vi "CRYTS Step Insert.vi"(10 "Steps":refnum<vi>, 11 "Tree Task SequenceIn":refnum<vi>) -> (3 "Tree Task Sequence Out":refnum<vi>)   [LabVIEW 2013]
uses:
  CRYSystem/Typedef Control/CRYStep.ctl
  CRYProject Editor Global.vi
  CRYMainGlobal.vi
panel:
  # "Insert new step into Project window."
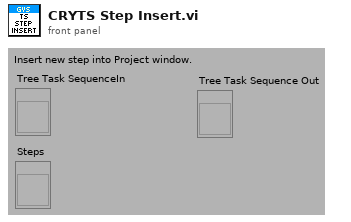
[diagram p1: front panel]
types:
  T1 = typedef "CRYTS.ctl" = cluster{"No.TS":u16, "TS File Path":path, "TS Name":string, "EditStepName":string, "Steps":T2[], "New State":bool, "Change State":bool, "Flattened CurveLib Data":string, "Document Data":string, "EditStepNo":u16, "Operator Start File":string, "Sequence Type":string, "Sequence Language":string}
  T2 = typedef "CRYStep.ctl" = cluster{"No.VI":i32, "Category":string, "StepName":string, "Seq setup flattened":string, "Comment":string, "Steps config.":bool[], "Jump config":i32[], "Start":dbl, "Increment":dbl, "Name":string, "Unit":string, "Y data":u16, "Y prefix":string, "Y dB ref":dbl, "Y unit":string, "Repeat State Array":cluster{"Start":dbl, "Increment":dbl, "Count":i32, "Num":i32}[]}
  T3 = cluster{"SourceRowNum":i32, "SourceCount":i32, "TargetRowNum":i32, "bResult":bool, "EditRowNum":i32}
  T4 = cluster{"Content":string, "Name":string, "Level":u32, "Category":string}[]
  T5 = cluster{"Content":string, "Name":string, "Level":u32, "Category":string}
  T6 = enum16{"Insert", "Remove", "Move up", "Move down"}
  T7 = cluster{"Start":dbl, "Increment":dbl, "Count":i32, "Num":i32}[]
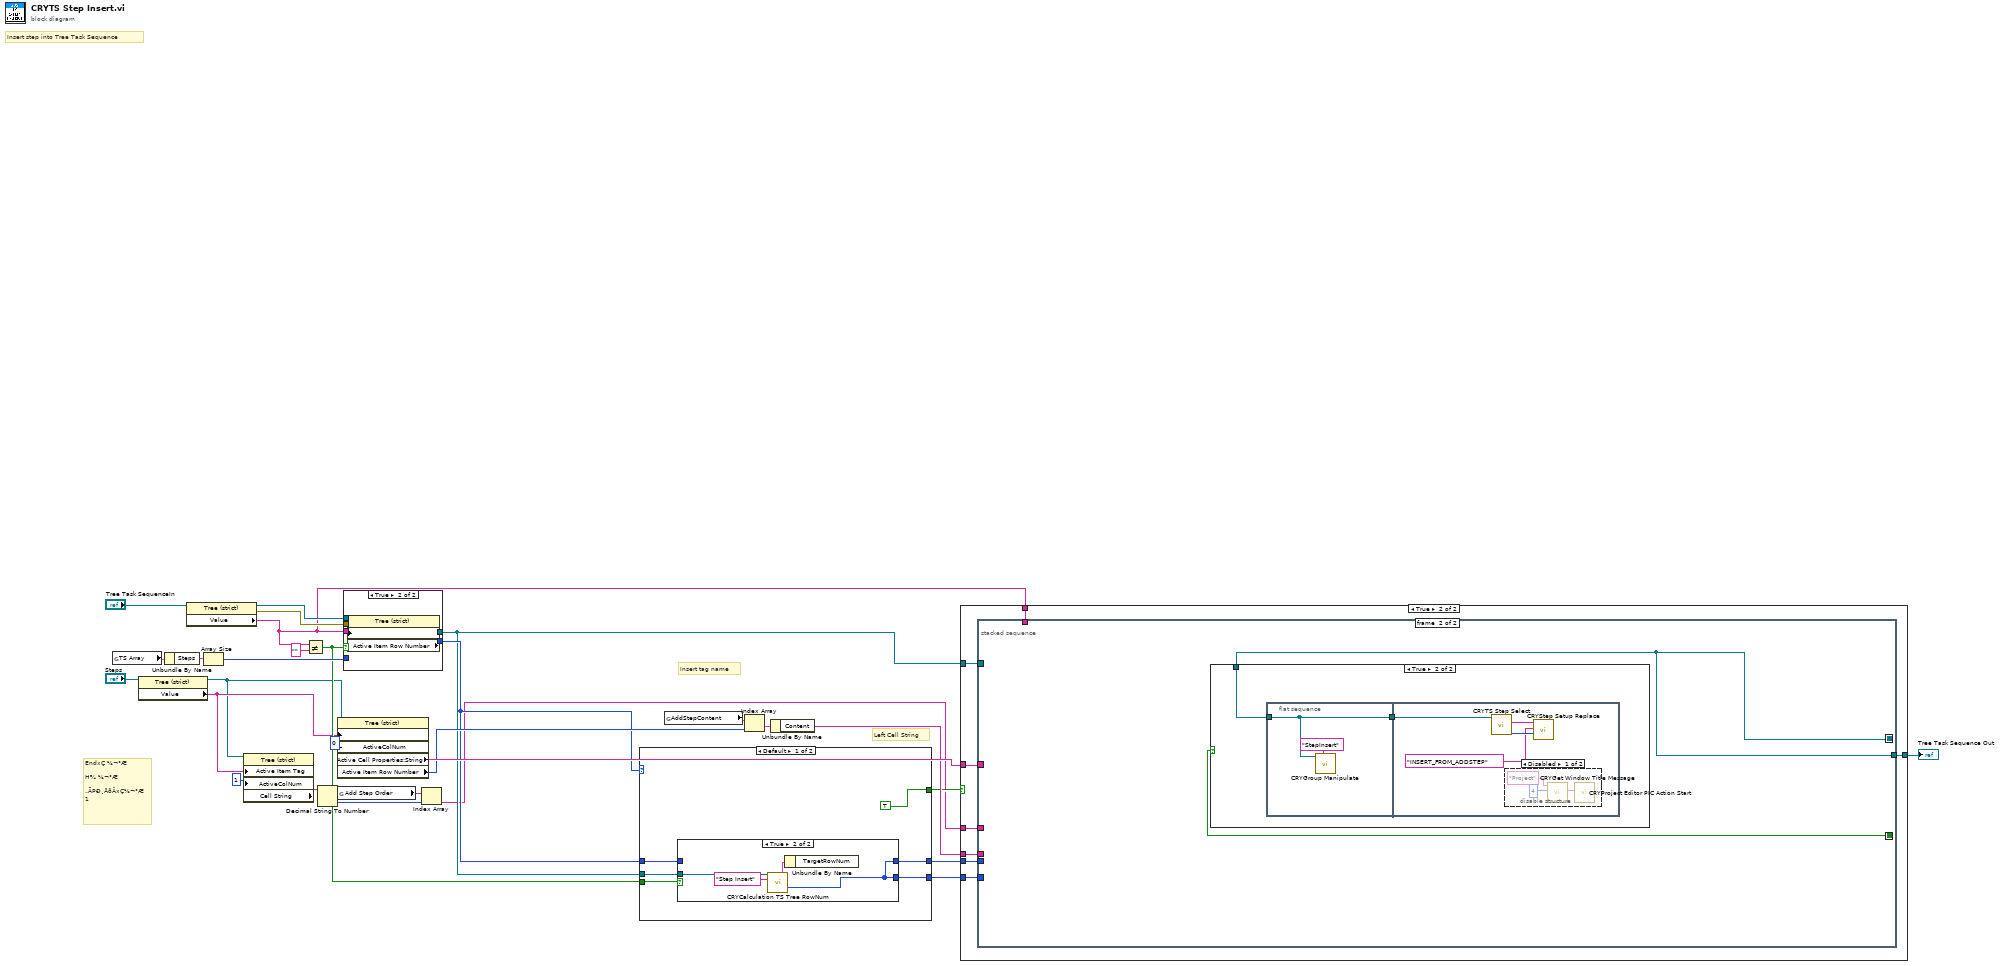
[diagram p0: block diagram]
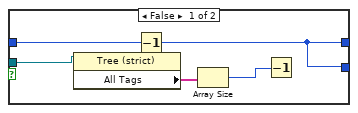
[diagram p2: hidden frame]
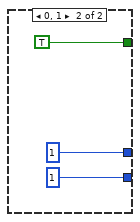
[diagram p3: hidden frame]
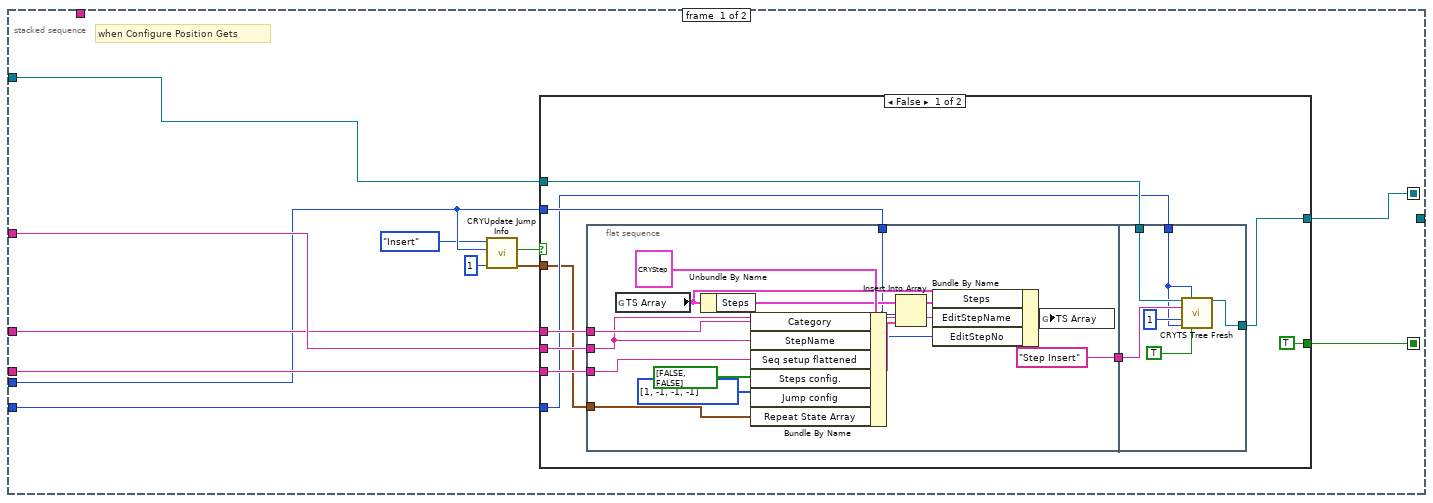
[diagram p5: hidden frame]
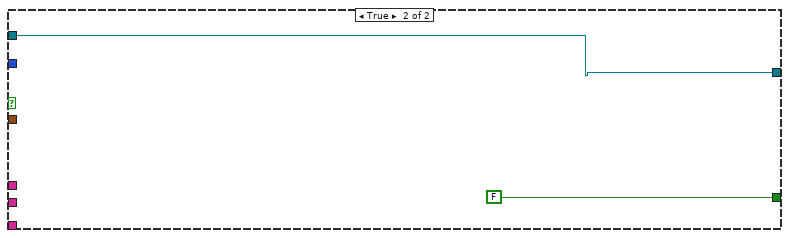
[diagram p6: hidden frame]
diagram:
  # "EndxÇ ½¬°Æ\n\nH¾ ½¬°Æ\n\n„ÃPÐ¸ÅðÄxÇ½¬°Æ\n1"
  # "Left Cell String"
  # "Insert tag name"
  # "Insert step into Tree Task Sequence"
  n1 = global read "CRYProject Editor Global.vi" "TS Array"() -> (w25:T1)
  n2 = property class="Tree (strict)"(reference="Steps") -> (reference out=w3:refnum<vi>, "Value"=w4:string)  [unwired: 1 in, 1 out]
  n3 = Unbundle By Name(w25) -> ("Steps"=w26:T2[])
  n4 = property class="Tree (strict)"(reference="Tree Task SequenceIn") -> (reference out=w24:refnum<vi>, error out=w23:errorcluster, "Value"=w10:string)  [unwired: 1 in]
  n5 = Array Size(array=w26) -> (size(s)=w13:i32)
  n6 = property class="Tree (strict)"(reference=w3, "Active Item Tag"=w4, "ActiveColNum"=1 ("Active Cell:Active Column Number")) -> ("Cell String"=w7:string)  [unwired: 1 in, 2 out]
  n7 = Not Equal?(x=w10, y="") -> (x != y?=w12:bool)
  n8 = Decimal String To Number(string=w7) -> (number=w5:i32)  [unwired: 2 in, 1 out]
  n9 = property class="Tree (strict)"(reference=w3, "Active Item Properties:Active Item (Tag)"=w4, "ActiveColNum"=0 ("Active Cell:Active Column Number")) -> ("Active Cell Properties:String"=w22:string, "Active Item Row Number"=w21:i32)  [unwired: 1 in, 2 out]
  n10 = global read "CRYMainGlobal.vi" "Add Step Order"() -> (w6:string[])
  n11 = case shown="True" w12 {
    tunnel: w23 -> [_ w36]
    tunnel: [w30 w35] -> w14
    tunnel: [w31 w34] -> w11
    tunnel: w10 -> [_ w33]
    tunnel: w24 -> [w31 w32]
    tunnel: w13 -> [w30 _]
    frame False {
    }
    frame True {
      n12 = property class="Tree (strict)"(reference=w32, error in=w36, "Active Item Properties:Active Item (Tag)"=w33) -> (reference out=w34:refnum<vi>, "Active Item Row Number"=w35:i32)  [unwired: 1 out]
    }
  }
  n13 = Index Array(array=w6, index=w5) -> (element=w2:string)
  n14 = case shown="Default" w14 {
    tunnel: [TRUE TRUE] -> w18
    tunnel: w14 -> [w38 _]
    tunnel: [w41 1 ("Active Item Row Number")] -> w15
    tunnel: w12 -> [w40 _]
    tunnel: w11 -> [w39 _]
    tunnel: [w37 1 ("Active Item Row Number")] -> w9
    frame Default {
      n15 = case shown="True" w40 {
        tunnel: w38 -> [w47 _]
        tunnel: [w43 w48] -> w41
        tunnel: w39 -> [w45 w51]
        tunnel: [w43 w48] -> w37
        frame False {
          n16 = property class="Tree (strict)"(reference=w45) -> ("All Tags"=w46:string[])  [unwired: 1 in, 2 out]
          n17 = Decrement(x=w47) -> (x-1=w43:i32)
          n18 = Array Size(array=w46) -> (size(s)=w44:i32)
          n19 = Decrement(x=w44) -> ()  [unwired: 1 out]
        }
        frame True {
          n20 = call "CRYCalculation TS Tree RowNum.vi"("Tree Task SequenceIn"=w51, "sOption"="Step Insert") -> ("DispInfo Cluster Out"=w49:T3, "TargetRowNum"=w48:i32)  [unwired: 7 in, 5 out]
          n21 = Unbundle By Name(w49) -> ()  [unwired: 1 out]
        }
      }
    }
    frame 0, 1 {
    }
  }
  n22 = global read "CRYProject Editor Global.vi" "AddStepContent"() -> (w17:T4)
  n23 = Index Array(array=w17, index=w21) -> (element=w16:T5)
  n24 = Unbundle By Name(w16) -> ("Content"=w19:string)
  n25 = case shown="True" w18 {
    tunnel: w11 -> [w55 w63]
    tunnel: w22 -> [_ w62]
    tunnel: w2 -> [_ w61]
    tunnel: w19 -> [_ w60]
    tunnel: [w55 w59] -> w29
    tunnel: w10 -> [_ w58]
    tunnel: w15 -> [_ w57]
    tunnel: w9 -> [_ w56]
    frame False {
    }
    frame True {
      n26 = stacked-sequence {
        seq-local: [w75 _] -> [_ w109]
        seq-local: [w70 _] -> [_ w108]
        tunnel: w63 -> [w74 _]
        tunnel: w62 -> [w73 _]
        tunnel: w61 -> [w72 _]
        tunnel: w60 -> [w71 _]
        tunnel: [_ w109] -> w59
        tunnel: w58 -> [_ _]
        tunnel: w57 -> [w69 _]
        tunnel: w56 -> [w68 _]
        frame #0 {
          # "when Configure Position Gets"
          n27 = call "CRYUpdate Jump Info.vi"("SourceCount"=1 ("Number of steps inserted"), "Step number Selected"=w69, "Action"=T6."Insert") -> ("Jump State Out"=w64:T7, "Canceled?"=w66:bool)  [unwired: 7 in]
          n28 = case shown="False" w66 {
            tunnel: [w80 w106] -> w75
            tunnel: w73 -> [w85 _]
            tunnel: w72 -> [w84 _]
            tunnel: w71 -> [w83 _]
            tunnel: w69 -> [w78 _]
            tunnel: [TRUE ("Jumps broken prev (F)") FALSE ("Jumps broken prev (F)")] -> w70
            tunnel: w74 -> [w81 w106]
            tunnel: w68 -> [w77 _]
            tunnel: w64 -> [w76 _]
            frame False {
              n29 = flat-sequence {
                tunnel: w85 -> [w88]
                tunnel: w84 -> [w99]
                tunnel: w83 -> [w98]
                tunnel: w78 -> [w89]
                tunnel: ["Step Insert" ("sOption")] -> w79
                tunnel: w76 -> [w86]
                tunnel: w81 -> [w105]
                tunnel: [w104] -> w80
                tunnel: w79 -> [w102]
                tunnel: w77 -> [w100]
                frame #0 {
                  n30 = global read "CRYProject Editor Global.vi" "TS Array"() -> (w92:T1)
                  n31 = Unbundle By Name(w92) -> ("Steps"=w93:T2[])
                  n32 = Bundle By Name(cluster=T2 {"No.VI"=0, "Category"="", "StepName"="", "Seq setup flattened"="", "Comment"="", "Steps config."=[], "Jump config"=[], "Start"=0.0, "Increment"=0.0, "Name"="", "Unit"="", "Y data"=0, "Y prefix"="", "Y dB ref"=0.0, "Y unit"="", "Repeat State Array"=[]} ("Step"), "Category"=w99, "StepName"=w88, "Seq setup flattened"=w98, "Steps config."=bool[] [FALSE, FALSE], "Jump config"=i32[] [1, -1, -1, -1], "Repeat State Array"=w86) -> (w97:T2)
                  n33 = Insert Into Array(array=w93, index=w89, new element=w97) -> (w90:T2[])
                  n34 = Bundle By Name(cluster=w92, "Steps"=w90, "EditStepName"=w88, "EditStepNo"=w89) -> (w91:T1)
                  n35 = global write "CRYProject Editor Global.vi" "TS Array"(w91) -> ()
                }
                frame #1 {
                  n36 = call "CRYTS Tree Fresh.vi"("SequenceTree"=w105, "Edit Index"=w100, "sOption"=w102, "SourceCount"=1, "Target Index"=w100, "Is Refresh?"=TRUE) -> ("SequenceTree out"=w104:refnum<vi>)  [unwired: 9 in]
                }
              }
            }
            frame True {
            }
          }
        }
        frame #1 {
          n37 = case shown="True" w108 {
            tunnel: w109 -> [_ w111]
            frame False {
            }
            frame True {
              n38 = flat-sequence {
                tunnel: w111 -> [w113]
                tunnel: [w113] -> w110
                tunnel: w110 -> [w117]
                frame #0 {
                  n39 = call "CRYGroup Manipulate.vi"("sAction"="StepInsert", "Tree in"=w113) -> ()  [unwired: 6 in, 4 out]
                }
                frame #1 {
                  n40 = call "CRYTS Step Select.vi"("Tree reference In"=w117) -> ("nData_Out"=w115:i32, "sData_Out"=w116:string)  [unwired: 9 out]
                  n41 = disable-structure shown="Disabled" {
                    frame Disabled {
                      n42 = call "CRYGet Window Title Message.vi"("No"=4 ("Error No"), "Kind"="Project") -> ("Unicode String"=w119:string)  [unwired: 4 in, 5 out]
                      n43 = call "CRYProject Editor PIC Action Start.vi"("sData"=w119) -> ()  [unwired: 11 in]
                    }
                    frame Enabled {
                    }
                  }
                  n44 = call "CRYStep Setup Replace.vi"("Current Step Setup VI No"=w115, "sOption"="INSERT_FROM_ADDSTEP", "Category"=w116) -> ()  [unwired: 1 in, 8 out]
                }
              }
            }
          }
        }
      }
    }
  }
  "Tree Task Sequence Out" <- w29
